vi "MDriveCommandDescriptors.vi"(4 "MDriveCommand":T2="DePowerMotor") -> (0 "Error":bool, 1 "CommandDescriptorOutput":T1)   [LabVIEW 2013]
uses:
  MDriveDriveCommand.ctl
  CommandDescriptor.ctl
  ~subVIs/CommandPhases.ctl
panel:
  in  "CommandDescriptorArray":T1[](array[typedef])=[{"Command"="Config", "Mnemonic"="<>", "Min"=nan, "Max"=nan, "ActionPath"=["PassCommand", "Communicate", "CheckEcho", "Done"]}, {"Command"="DePowerMotor", "Mnemonic"="DE", "Min"=0.0, "Max"=1.0, "ActionPath"=["CheckLimits", "AssembleCommand", "Communicate", "CheckEcho", "AssembleReadback", "Communicate", "ParseNumber", "Done"]}, {"Command"="StopEmergency", "Mnemonic"="\u0005", "Min"=nan, "Max"=nan, "ActionPath"=["PassCommand", "Communicate", "CheckEcho", "Done"]}, {"Command"="StopGently", "Mnemonic"="SL 0", "Min"=nan, "Max"=nan, "ActionPath"=["PassCommand", "Communicate", "CheckEcho", "Done"]}, {"Command"="GoNow", "Mnemonic"="MA R1", "Min"=nan, "Max"=nan, "ActionPath"=["PassCommand", "Communicate", "Done"]}, {"Command"="AccelerationSet", "Mnemonic"="A", "Min"=0.0, "Max"=61035160.0, "ActionPath"=["CheckLimits", "AssembleCommand", "Communicate", "CheckEcho", "AssembleReadback", "Communicate", "ParseNumber", "DecelerationSet", "Done"]}, {"Command"="VelocitySet", "Mnemonic"="VM", "Min"=0.0, "Max"=5000000.0, "ActionPath"=["CheckLimits", "AssembleCommand", "Communicate", "CheckEcho", "AssembleReadback", "Communicate", "ParseNumber", "Done"]}, {"Command"="PositionSetTarget", "Mnemonic"="R1", "Min"=-2147483648.0, "Max"=2147483647.0, "ActionPath"=["CheckLimits", "AssembleCommand", "Communicate", "CheckEcho", "AssembleReadback", "Communicate", "ParseNumber", "Done"]}, {"Command"="PositionReadEncoderPulses", "Mnemonic"="PR C2", "Min"=nan, "Max"=nan, "ActionPath"=["PassCommand", "Communicate", "ParseNumber", "Done"]}, {"Command"="PositionReadMotorPulses", "Mnemonic"="PR C1", "Min"=nan, "Max"=nan, "ActionPath"=["PassCommand", "Communicate", "ParseNumber", "Done"]}, {"Command"="DecelerationSet", "Mnemonic"="D", "Min"=0.0, "Max"=61035200.0, "ActionPath"=["CheckLimits", "AssembleCommand", "Communicate", "CheckEcho", "AssembleReadback", "Communicate", "ParseNumber", "Done"]}, {"Command"="GetError", "Mnemonic"="PR ER", "Min"=nan, "Max"=nan, "ActionPath"=["PassCommand", "Communicate", "ParseError", "Done"]}, {"Command"="IsMoving", "Mnemonic"="PR MV", "Min"=nan, "Max"=nan, "ActionPath"=["PassCommand", "Communicate", "ParseNumber", "Done"]}, {"Command"="LiveVelocityControl", "Mnemonic"="SL", "Min"=-300.0, "Max"=300.0, "ActionPath"=["CheckLimits", "AssembleCommand", "Communicate", "CheckEcho", "Done"]}]
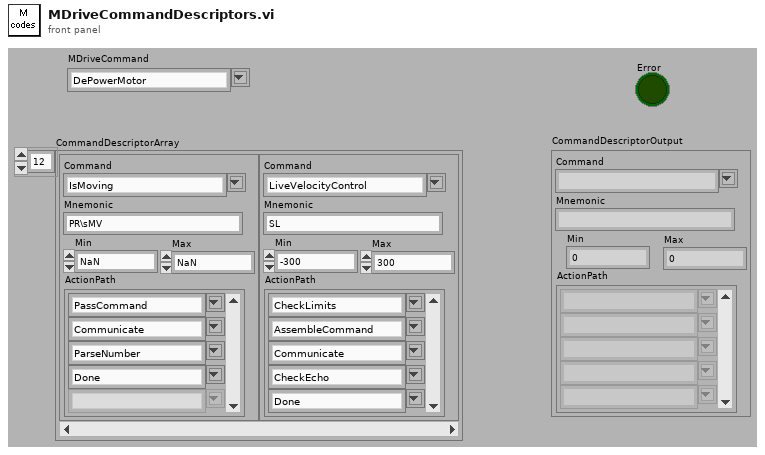
[diagram p1: front panel]
types:
  T1 = typedef "CommandDescriptor.ctl" = cluster{"Command":T2, "Mnemonic":string, "Min":dbl, "Max":dbl, "ActionPath":T3[]}
  T2 = typedef "MDriveDriveCommand.ctl" = string
  T3 = typedef "CommandPhases.ctl" = string
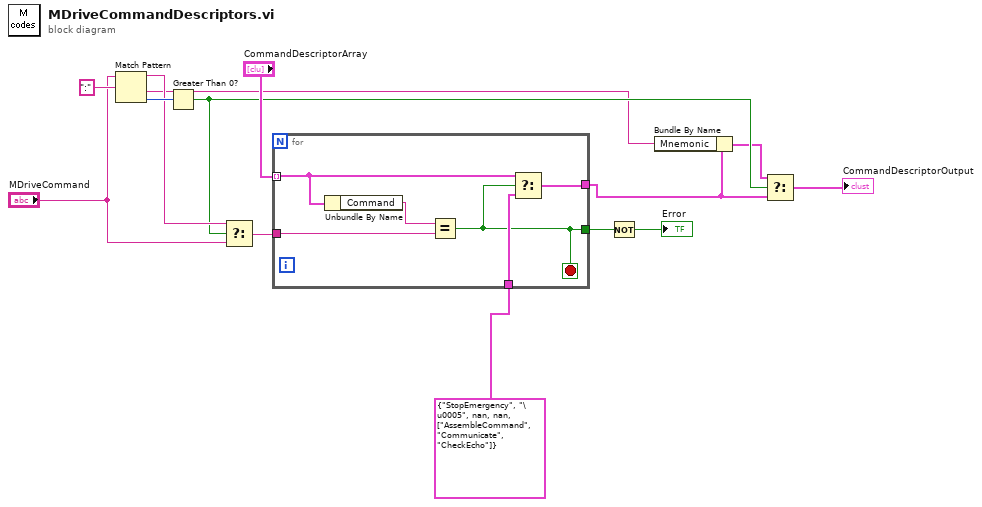
[diagram p0: block diagram]
diagram:
  n1 = Match Pattern(string="MDriveCommand", regular expression=":") -> (before substring=w6:T2, after substring=w1:T2, offset past match=w9:i32)  [unwired: 2 out]
  n2 = Greater Than 0?(x=w9) -> (x > 0?=w4:bool)
  n3 = Select(t=w6, s=w4, f="MDriveCommand") -> (s? t:f=w8:T2)
  n4 = for {
    tunnel: "CommandDescriptorArray" -> [w17] mode=indexing
    tunnel: w8 -> [w19]
    tunnel: [w18] -> w3
    tunnel: T1 {"Command"="StopEmergency", "Mnemonic"="\u0005", "Min"=nan, "Max"=nan, "ActionPath"=["AssembleCommand", "Communicate", "CheckEcho"]} ("CommandDescriptorOutput") -> [w16]
    tunnel: [w15] -> w13
    stop <- w15 stop-if-true
    n5 = Unbundle By Name(w17) -> ("Command"=w20:T2)
    n6 = Equal?(x=w20, y=w19) -> (x = y?=w15:bool)
    n7 = Select(t=w17, s=w15, f=w16) -> (s? t:f=w18:T1)
  }
  n8 = Not(x=w13) -> (.not. x?=→"Error":bool)
  n9 = Bundle By Name(cluster=w3, "Mnemonic"=w1) -> (w2:T1)
  n10 = Select(t=w2, s=w4, f=w3) -> (s? t:f=→"CommandDescriptorOutput":T1)
